vi "Write Executions.vi"(8 "error in (no error)":errorcluster, 10 "Executions":refnum<data-value>[](array[refnum]), 11 "Application in":refnum<class "Application.lvclass">) -> (0 "error out":errorcluster, 3 "Application out":refnum<class "Application.lvclass">)   [LabVIEW 2015, in "Application.lvclass"]
uses:
  Application.lvclass
  Execution.lvclass
  Application.lvclass/Application.ctl
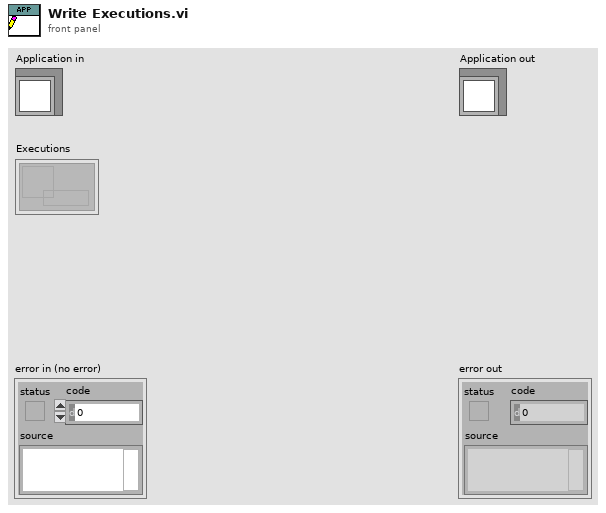
[diagram p1: front panel]
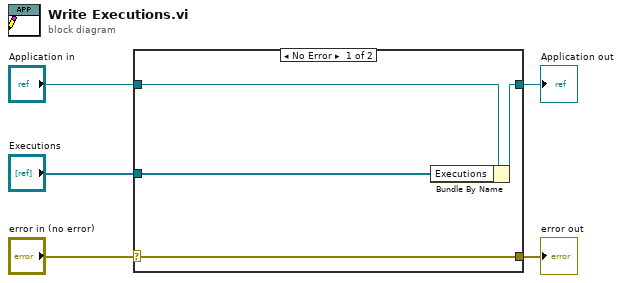
[diagram p0: block diagram]
diagram:
  n1 = case shown="No Error" "error in (no error)" {
    selector: "error in (no error)" -> [w9 w10]
    tunnel: [w9 w10] -> w4
    tunnel: [w7 w11] -> w2
    tunnel: "Application in" -> [w8 w11]
    tunnel: "Executions" -> [w6 _]
    frame No Error {
      n2 = Bundle By Name(cluster=w8, "Executions"=w6) -> (w7:refnum<class "Application.lvclass">)
    }
    frame Error {
    }
  }
  "error out" <- w4
  "Application out" <- w2
